vi "NTViewerUI.vi"(10 "Plugin Info":T1, 11 "Tree Control Format String (*)":string="*") -> ()   [LabVIEW 2016]
uses:
  General/CorePluginInfo.ctl
  General/CoreDashGlobal.vi
panel:
  in  "Tab Control":enum32{"All Table Entries", "User 1"}(tab)
  in  "NT Entries":string(tree)
  out "IntakeWheels_Output":dbl(slide) scale=-1.0..1.0 scale format="%#_7g"
  out "ChooChoo_PID_Enabled":bool
  out "IntakeLift_PID_Enabled":bool
  out "ChooChoo_Setpoint":dbl
  out "ChooChoo_Zeroed":bool
  out "ChooChoo_Output":dbl(slide) scale=-1.0..1.0 scale format="%#_7g"
  out "ChooChoo_Position":dbl
  out "IntakeLift_Setpoint":dbl
  out "IntakeLift_Zeroed":bool
  out "IntakeLift_Output":dbl(slide) scale=-1.0..1.0 scale format="%#_7g"
  out "IntakeLift_Position":dbl
  # "First page of user controls. Here you can add as many controls as you like, as well as create other pages\nfor controls. These will all automatically be bound to the SmartDashboard."
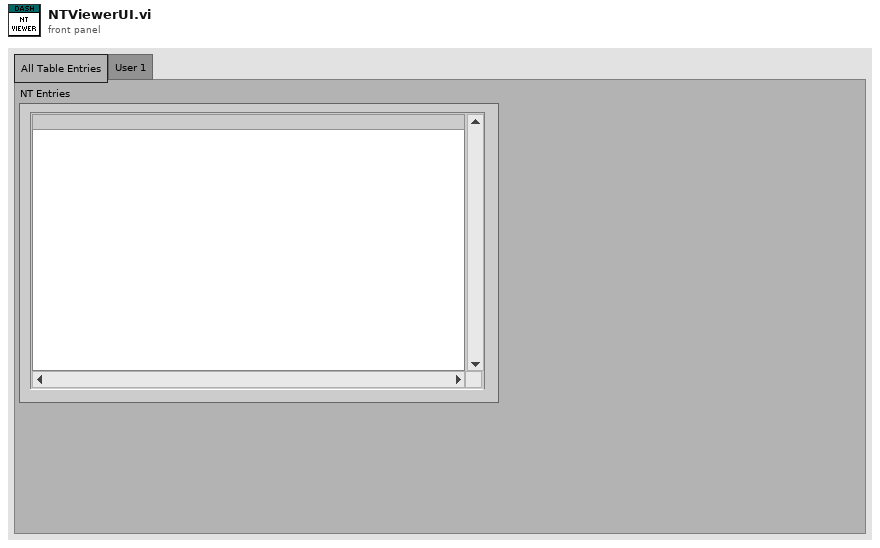
[diagram p1: front panel]
types:
  T1 = typedef "CorePluginInfo.ctl" = cluster{"Notifiers":cluster{"Robot IP Notifier":refnum<notifier>, "Window Mode Notifier":refnum<notifier>, "Stop Notifier":refnum<notifier>}}
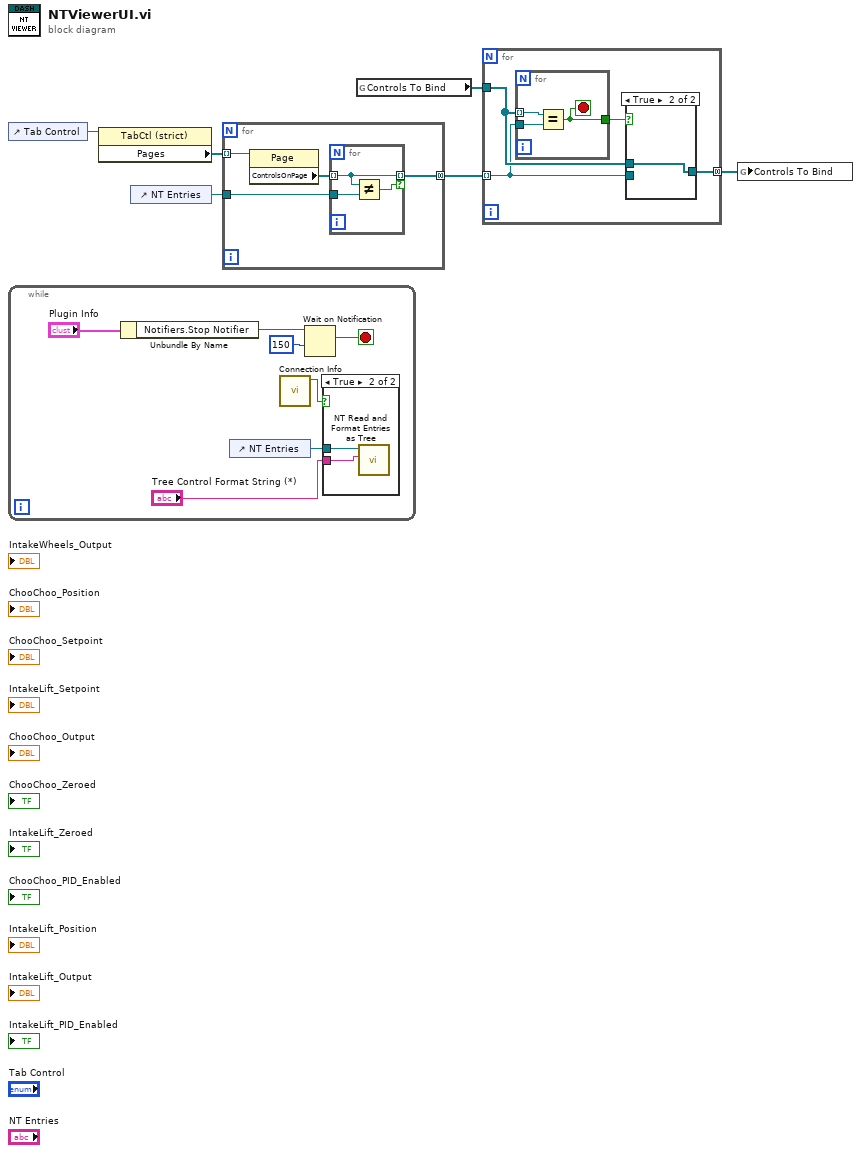
[diagram p0: block diagram]
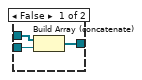
[diagram p3: hidden frame]
diagram:
  n1 = control-ref of="Tab Control"() -> (w4:refnum<vi>)
  n2 = while {
    stop <- w11 stop-if-true
    n3 = Unbundle By Name("Plugin Info") -> ("Notifiers.Stop Notifier"=w12:refnum<notifier>)
    n4 = control-ref of="NT Entries"() -> (w8:refnum<vi>)
    n5 = call <vilib>:"Connection Info.vi"() -> ("Connected"=w9:bool)  [unwired: 10 in, 1 out]
    n6 = Wait on Notification(notifier=w12, timeout in ms (-1)=150) -> (notification=w11:bool)  [unwired: 2 in, 3 out]
    n7 = case shown="True" w9 {
      tunnel: w8 -> [_ w15]
      tunnel: "Tree Control Format String (*)" -> [_ w14]
      frame False {
      }
      frame True {
        n8 = call <vilib>:"NT Read and Format Entries as Tree.vi"("Name Pattern"=w14, "Tree Refnum"=w15) -> ()  [unwired: 8 in, 2 out]
      }
    }
  }
  n9 = property class="TabCtl (strict)"(reference=w4) -> ("Pages"=w5:refnum<vi>[])  [unwired: 1 in, 2 out]
  n10 = control-ref of="NT Entries"() -> (w6:refnum<vi>)
  n11 = for {
    tunnel: w5 -> [w19] mode=indexing
    tunnel: w6 -> [w18]
    tunnel: [w16] -> w2 mode=concatenating
    n12 = property class="Page"(reference=w19) -> ("ControlsOnPage"=w17:refnum<vi>[])  [unwired: 1 in, 2 out]
    n13 = for {
      tunnel: w17 -> [w21] mode=indexing
      tunnel: w18 -> [w22]
      tunnel: [w21] -> w16 mode=indexing if=w20
      n14 = Not Equal?(x=w21, y=w22) -> (x != y?=w20:bool)
    }
  }
  n15 = global read "CoreDashGlobal.vi" "Controls To Bind"() -> (w3:refnum<vi>[])
  n16 = for {
    tunnel: w3 -> [w25]
    tunnel: w2 -> [w24] mode=indexing
    tunnel: [w23] -> w1 mode=concatenating
    n17 = for {
      tunnel: w25 -> [w32] mode=indexing
      tunnel: w24 -> [w33]
      tunnel: [w31] -> w26
      stop <- w31 stop-if-true
      n18 = Equal?(x=w32, y=w33) -> (x = y?=w31:bool)
    }
    n19 = case shown="True" w26 {
      tunnel: w25 -> [w29 w30]
      tunnel: w24 -> [w28 _]
      tunnel: [w27 w30] -> w23
      frame False {
        n20 = Build Array (concatenate)(w29, w28) -> (w27:refnum<vi>[])
      }
      frame True {
      }
    }
  }
  n21 = global write "CoreDashGlobal.vi" "Controls To Bind"(w1) -> ()
